vi "Messenger.vi"() -> ()   [LabVIEW 2019]
uses:
  #cluster_ApplicationData.ctl
panel:
  in  "My Port":u16=60056
  in  "Friend Port":u16=60055
  out "Connected?":bool
  in  "Friend IP Address":string="10.8.3.120"
  out "Chat":string[](array[string])
  in  "Message":string
  in  "Send":bool
  in  "Stop":bool
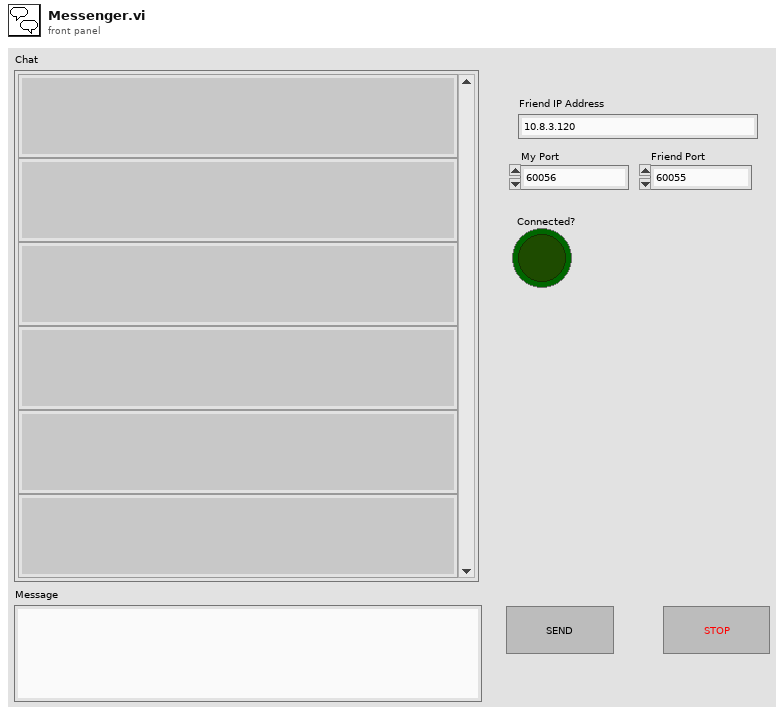
[diagram p1: front panel]
types:
  T1 = typedef "#cluster_ApplicationData.ctl" = cluster{"Connected?":bool, "Chat":string[], "connection ID":refnum<k5>}
  T2 = enum16{"Standard", "Buffered", "CRLF", "Immediate"}
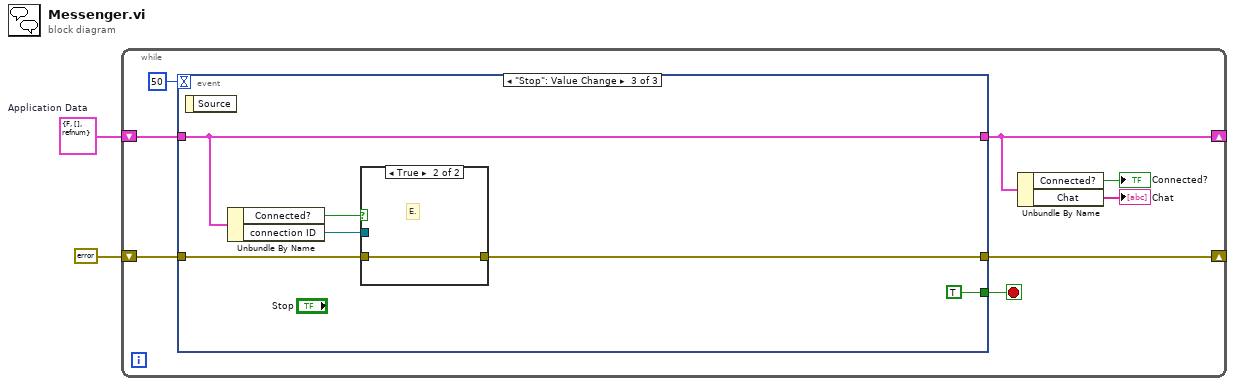
[diagram p0: block diagram]
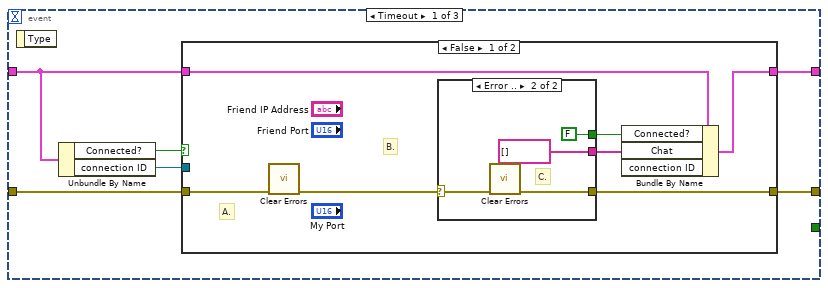
[diagram p2: hidden frame]
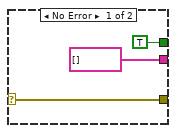
[diagram p3: hidden frame]
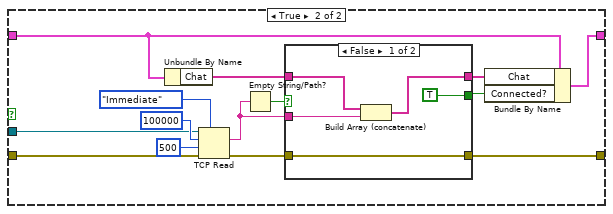
[diagram p4: hidden frame]
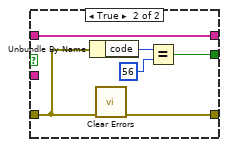
[diagram p5: hidden frame]
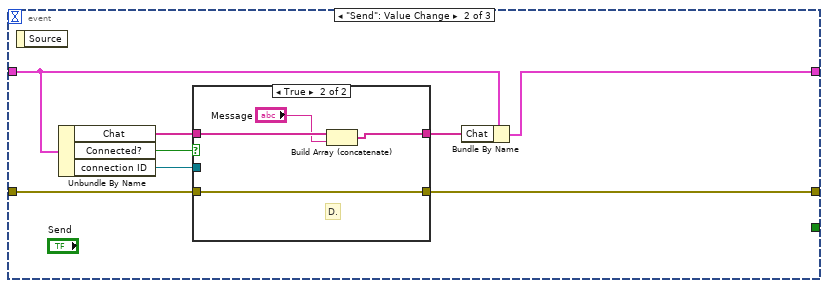
[diagram p6: hidden frame]
diagram:
  w1 = T1 {"Connected?"=FALSE, "Chat"=[], "connection ID"=refnum}  # Application Data
  n1 = while {
    shift-right: [w9] -> _
    shift-left: errorcluster {"status"=FALSE, "code"=0, "source"=""} ("error out") -> [w8]
    shift-right: [w6] -> _
    shift-left: w1 -> [w7]
    stop <- w3 stop-if-true
    n2 = event shown="[2] \"Stop\": Value Change" {
      selector: _ -> [_ _ _]
      dyn-events: _ -> [_ _ _]
      timeout: 50 -> [_ _ _]
      tunnel: [_ _ TRUE ("stop")] -> w3
      tunnel: [w15 w62 w73] -> w9
      tunnel: w8 -> [w16 w63 w74]
      tunnel: w7 -> [w14 w58 w70]
      tunnel: [w12 w56 w70] -> w6
      event Timeout {
        n3 = event-data() -> ()  [unwired: 1 in, 1 out]
        n4 = Unbundle By Name(w14) -> ("Connected?"=w13:bool, "connection ID"=w11:refnum<k5>)
        n5 = case shown="False" w13 {
          tunnel: w16 -> [w18 w44]
          tunnel: [w23 w42] -> w15
          tunnel: w14 -> [w22 w35]
          tunnel: [w19 w32] -> w12
          tunnel: w11 -> [_ w31]
          frame False {
            # "B."
            # "A."
            n6 = call <vilib>:"Clear Errors.vi"("error in (no error)"=w18) -> ("error out"=w17:errorcluster)  [unwired: 5 in, 1 out]
            n7 = case shown="Error .." w17 {
              selector: w17 -> [w25 w30]
              tunnel: [w25 w29] -> w23
              tunnel: [TRUE ("Connected?") FALSE ("Connected?")] -> w21
              tunnel: [string[] [] string[] []] -> w20
              frame No Error {
              }
              frame Error {
                # "C."
                n8 = call <vilib>:"Clear Errors.vi"("error in (no error)"=w30) -> ("error out"=w29:errorcluster)  [unwired: 5 in, 1 out]
              }
            }
            n9 = Bundle By Name(cluster=w22, "Connected?"=w21, "Chat"=w20) -> (w19:T1)  [unwired: 1 in]
          }
          frame True {
            n10 = Unbundle By Name(w35) -> ("Chat"=w34:string[])
            n11 = TCP Read(connection ID=w31, bytes to read=100000, error in (no error)=w44, 7:T2."Immediate" ("mode (standard)"), 9:500 ("timeout ms (25000)")) -> (data out=w41:string, error out=w39:errorcluster)  [unwired: 1 out]
            n12 = Empty String/Path?(string/path=w41) -> (empty?=w40:bool)
            n13 = case shown="False" w40 {
              tunnel: w41 -> [w49 _]
              tunnel: [w46 w55] -> w42
              tunnel: [TRUE w50] -> w36
              tunnel: w39 -> [w46 w53]
              tunnel: w34 -> [w47 w54]
              tunnel: [w45 w54] -> w33
              frame False {
                n14 = Build Array (concatenate)(w47, w49) -> (w45:string[])
              }
              frame True {
                n15 = Unbundle By Name(w53) -> ("code"=w52:i32)
                n16 = call <vilib>:"Clear Errors.vi"("error in (no error)"=w53) -> ("error out"=w55:errorcluster)  [unwired: 5 in, 1 out]
                n17 = Equal?(x=w52, y=56) -> (x = y?=w50:bool)
              }
            }
            n18 = Bundle By Name(cluster=w35, "Chat"=w33, "Connected?"=w36) -> (w32:T1)
          }
        }
      }
      event "Send": Value Change {
        n19 = event-data() -> ()  [unwired: 1 in, 1 out]
        n20 = Unbundle By Name(w58) -> ("Chat"=w60:string[], "Connected?"=w61:bool, "connection ID"=w59:refnum<k5>)
        n21 = case shown="True" w61 {
          tunnel: w63 -> [w65 w69]
          tunnel: w59 -> [_ _]
          tunnel: [w65 w69] -> w62
          tunnel: w60 -> [w64 w68]
          tunnel: [w64 w66] -> w57
          frame False {
          }
          frame True {
            # "D."
            n22 = Build Array (concatenate)(w68, "Message") -> (w66:string[])
          }
        }
        n23 = Bundle By Name(cluster=w58, "Chat"=w57) -> (w56:T1)
      }
      event "Stop": Value Change {
        n24 = event-data() -> ()  [unwired: 1 in, 1 out]
        n25 = Unbundle By Name(w70) -> ("Connected?"=w72:bool, "connection ID"=w71:refnum<k5>)
        n26 = case shown="True" w72 {
          tunnel: w74 -> [w76 w77]
          tunnel: w71 -> [_ _]
          tunnel: [w76 w77] -> w73
          frame False {
          }
          frame True {
            # "E."
          }
        }
      }
    }
    n27 = Unbundle By Name(w6) -> ("Connected?"=→"Connected?":bool, "Chat"=→"Chat":string[])
  }
